vi "Read SEQ.vi"(8 "error in (no error)":errorcluster, 11 "ObserverRegistry.lvclass in":refnum<class "ObserverRegistry.lvclass">) -> (0 "error out":errorcluster, 2 "SEQ":refnum<queue>, 3 "ObserverRegistry.lvclass out":refnum<class "ObserverRegistry.lvclass">)   [LabVIEW 2011, in "Messenging.lvlib" / "ObserverRegistry.lvclass"]
uses:
  ObserverRegistry.lvclass
  ObserverRegistryData.ctl
  Interprocess Messenger/SendOnly/Observer.lvclass
  ObserverRegistry.lvclass/ObserverRegistry.ctl
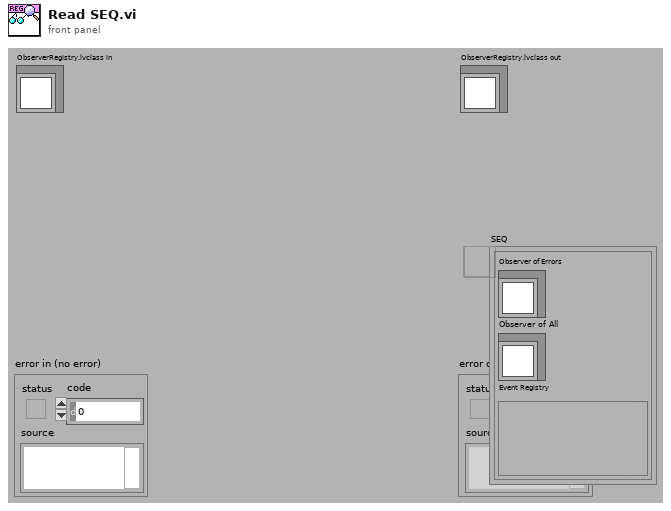
[diagram p1: front panel]
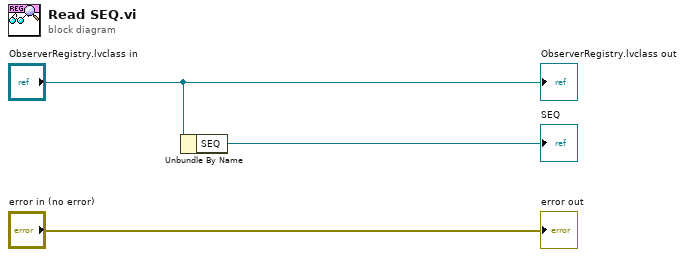
[diagram p0: block diagram]
diagram:
  n1 = Unbundle By Name("ObserverRegistry.lvclass in") -> ("SEQ"=→"SEQ":refnum<queue>)
  "error out" <- "error in (no error)"
  "ObserverRegistry.lvclass out" <- "ObserverRegistry.lvclass in"
